vi "input (SubVI).vi"(11 "Controller_NUC":sgl[](array[numeric])) -> (3 "Controller Input":T1 {"Joy1 Y-axis" scale=-32767.0..32767.0; "Joy2 Y-axis" scale=-32767.0..32767.0; "Joy2 X-axis" scale=-32767.0..32767.0; "Joy1 X-axis" scale=-32767.0..32767.0; "Z axis - LT~RT" scale=-32767.0..32767.0; "DPad" scale=0.0..360.0})   [LabVIEW 2016]
uses:
  YSH_XBOX360_joystick.ctl
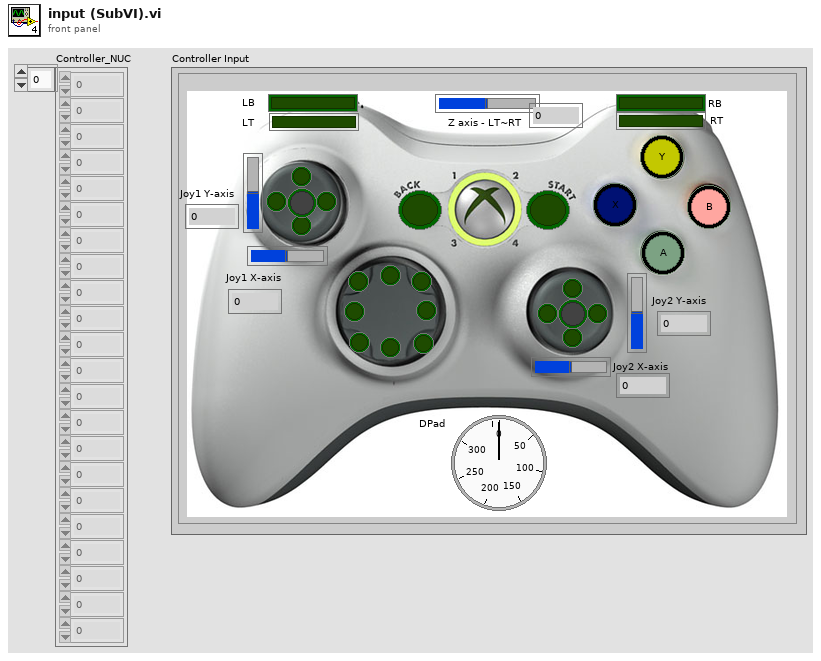
[diagram p1: front panel]
types:
  T1 = typedef "YSH_XBOX360_joystick.ctl" = cluster{"RR":bool, "RL":bool, "RD":bool, "RU":bool, "LR":bool, "LL":bool, "LD":bool, "LU":bool, "Back":bool, "Start":bool, "DPad":dbl, "D Pad":cluster{"0":bool, "45":bool, "90":bool, "135":bool, "180":bool, "215":bool, "270":bool, "315":bool}, "A":bool, "B":bool, "X":bool, "Y":bool, "LB":bool, "RB":bool, "LT":bool, "RT":bool, "Left Joy Push":bool, "Right Joy Push":bool, "Z axis - LT~RT":i32, "Joy1 X-axis":i32, "Joy2 X-axis":i32, "Joy2 Y-axis":i32, "Joy1 Y-axis":i32}
  T2 = cluster{"[0]":bool, "[1]":bool, "[2]":bool, "[3]":bool, "[4]":bool, "[5]":bool, "[6]":bool, "[7]":bool}
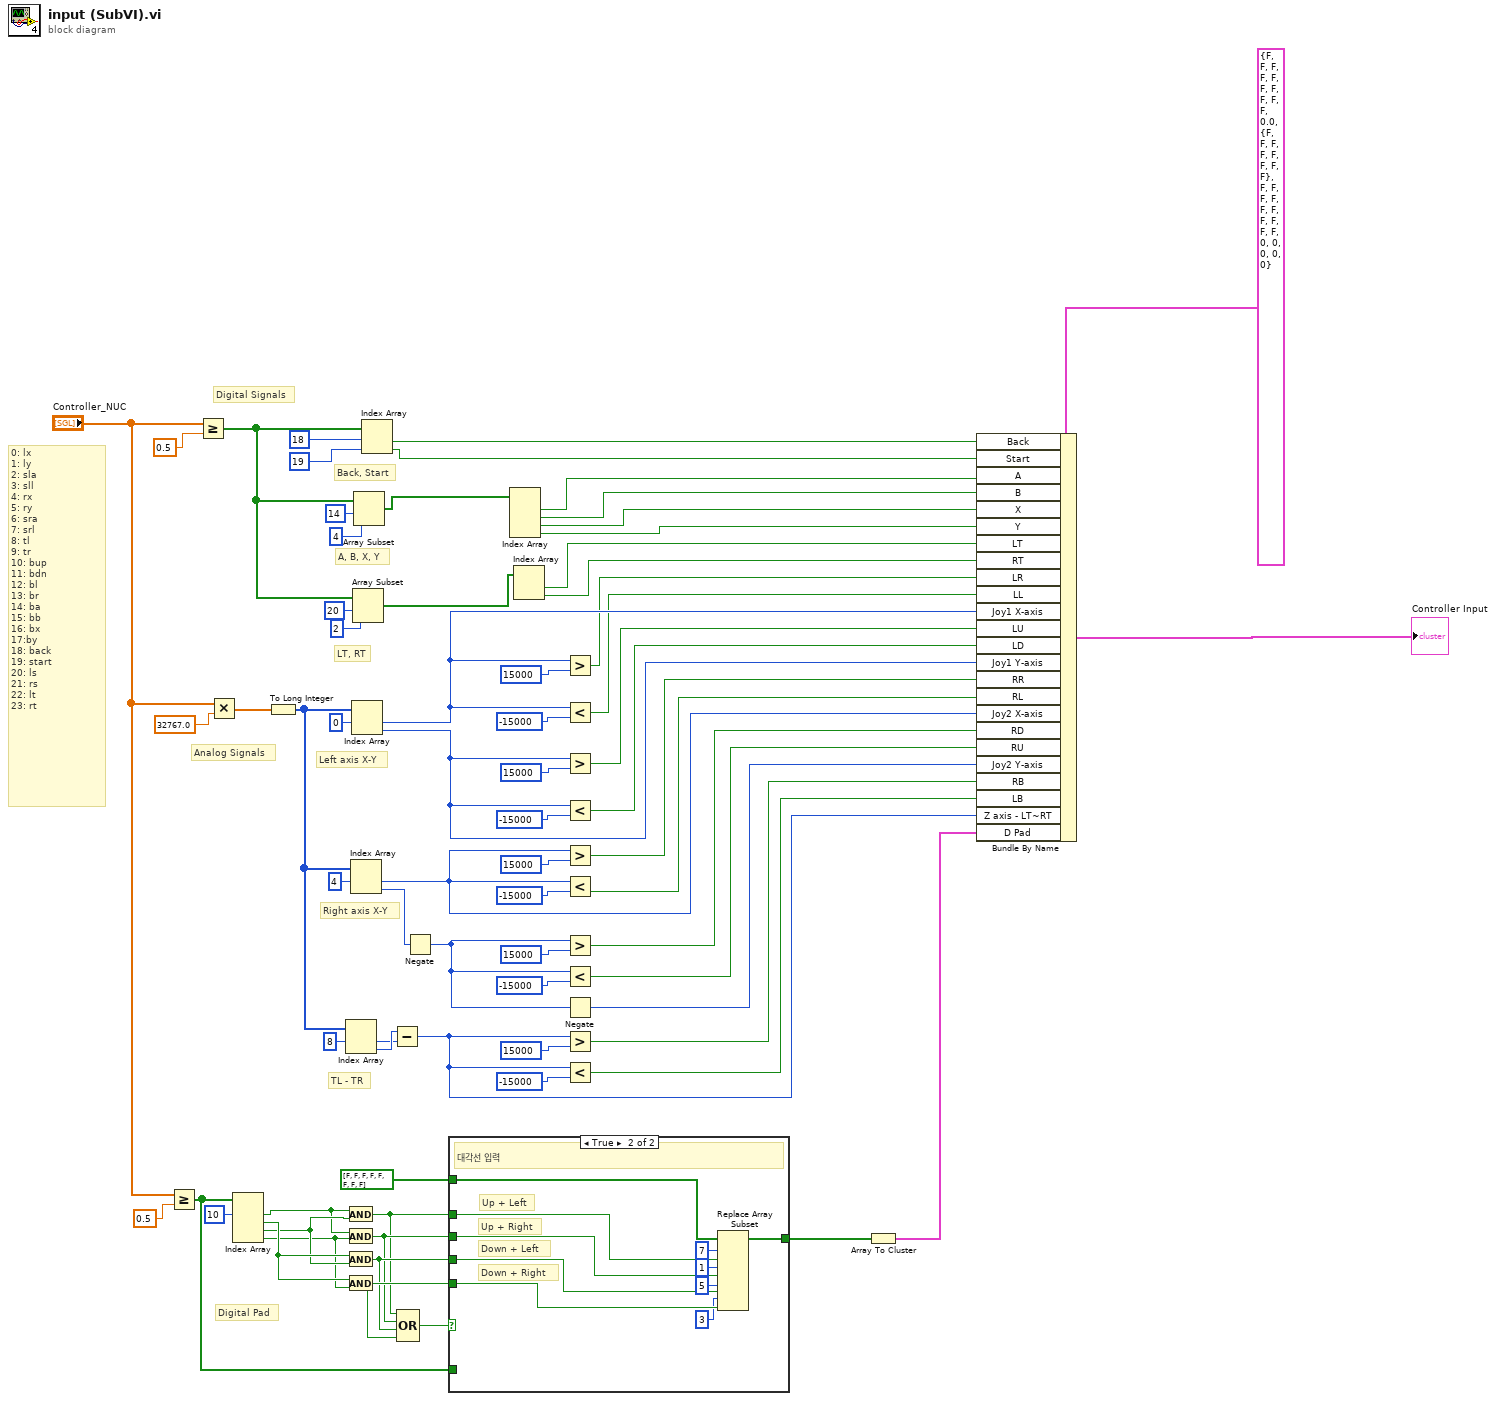
[diagram p0: block diagram]
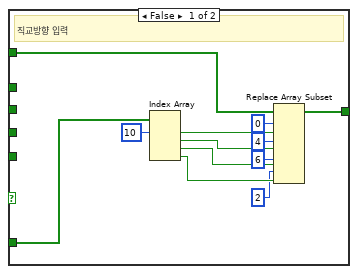
[diagram p2: hidden frame]
diagram:
  # "Analog Signals"
  # "Digital Pad"
  # "TL - TR"
  # "Right axis X-Y"
  # "Left axis X-Y"
  # "LT, RT"
  # "A, B, X, Y"
  # "Back, Start"
  # "Digital Signals"
  # "0: lx\n1: ly\n2: sla\n3: sll\n4: rx\n5: ry\n6: sra\n7: srl\n8: tl\n9: tr\n10: bup\n11: bdn\n12: bl\n13: br\n14: ba\n15: bb\n16: bx\n17:by\n18: back\n19: start\n20: ls\n21: rs\n22: lt\n23: rt"
  n1 = Greater Or Equal?(x="Controller_NUC", y=sgl 0.5) -> (x >= y?=w59:bool[])
  n2 = Greater Or Equal?(x="Controller_NUC", y=sgl 0.5) -> (x >= y?=w13:bool[])
  n3 = Multiply(x="Controller_NUC", y=sgl 32767.0) -> (x*y=w22:sgl[])
  n4 = Index Array(array=w59, index #1=10 ("인덱스")) -> (element #1=w68:bool, element #2=w71:bool, element #3=w70:bool, element #4=w69:bool)  [unwired: 3 in]
  n5 = To Long Integer(number=w22) -> (32bit integer=w48:i32[])
  n6 = Index Array(array=w48, index #1=8 ("인덱스")) -> (element #1=w49:i32, element #2=w50:i32)  [unwired: 1 in]
  n7 = And(x=w68, y=w70) -> (x .and. y?=w61:bool)
  n8 = And(x=w68, y=w69) -> (x .and. y?=w62:bool)
  n9 = And(x=w71, y=w70) -> (x .and. y?=w63:bool)
  n10 = And(x=w71, y=w69) -> (x .and. y?=w64:bool)
  n11 = Index Array(array=w48, index #1=4 ("인덱스")) -> (element #1=w41:i32, element #2=w42:i32)  [unwired: 1 in]
  n12 = Index Array(array=w48, index #1=0 ("인덱스")) -> (element #1=w28:i32, element #2=w33:i32)  [unwired: 1 in]
  n13 = Array Subset(array=w13, index=20 ("인덱스"), length=2 ("길이")) -> (w16:bool[])
  n14 = Array Subset(array=w13, index=14 ("인덱스"), length=4 ("길이")) -> (w8:bool[])
  n15 = Index Array(array=w13, index #1=18 ("인덱스"), index #2=19 ("인덱스")) -> (element #1=w3:bool, element #2=w4:bool)
  n16 = Subtract(x=w50, y=w49) -> (x-y=w55:i32)
  n17 = Compound Arithmetic op=OR(w61, w62, w63, w64) -> (w60:bool)
  n18 = Negate(x=w42) -> (-x=w45:i32)
  n19 = case shown="True" w60 {
    tunnel: bool[] [FALSE, FALSE, FALSE, FALSE, FALSE, FALSE, FALSE, FALSE] -> [w83 w93]
    tunnel: [w82 w92] -> w66
    tunnel: w59 -> [w80 _]
    tunnel: w61 -> [_ w91]
    tunnel: w62 -> [_ w90]
    tunnel: w63 -> [_ w89]
    tunnel: w64 -> [_ w88]
    frame False {
      # "직교방향 입력"
      n20 = Index Array(array=w80, index #1=10 ("인덱스")) -> (element #1=w79:bool, element #2=w78:bool, element #3=w77:bool, element #4=w76:bool)  [unwired: 3 in]
      n21 = Replace Array Subset(array=w83, new element #1=w79, index #1=0 ("인덱스"), new element #2=w78, index #2=4 ("인덱스"), new element #3=w77, index #3=6 ("인덱스"), new element #4=w76, index #4=2 ("인덱스")) -> (w82:bool[])
    }
    frame True {
      # "Up + Right"
      # "Down + Right"
      # "Down + Left"
      # "Up + Left"
      # "대각선 입력"
      n22 = Replace Array Subset(array=w93, new element #1=w91, index #1=7 ("인덱스"), new element #2=w90, index #2=1 ("인덱스"), new element #3=w89, index #3=5 ("인덱스"), new element #4=w88, index #4=3 ("인덱스")) -> (w92:bool[])
    }
  }
  n23 = Index Array(array=w8) -> (element #1=w9:bool, element #2=w10:bool, element #3=w11:bool, element #4=w12:bool)  [unwired: 4 in]
  n24 = Index Array(array=w16) -> (element #1=w17:bool, element #2=w18:bool)  [unwired: 2 in]
  n25 = Greater?(x=w28, y=15000) -> (0:w26:bool)
  n26 = Less?(x=w28, y=-15000) -> (x < y?=w27:bool)
  n27 = Greater?(x=w33, y=15000) -> (0:w31:bool)
  n28 = Less?(x=w33, y=-15000) -> (x < y?=w32:bool)
  n29 = Greater?(x=w41, y=15000) -> (0:w39:bool)
  n30 = Less?(x=w41, y=-15000) -> (x < y?=w40:bool)
  n31 = Greater?(x=w45, y=15000) -> (0:w43:bool)
  n32 = Less?(x=w45, y=-15000) -> (x < y?=w44:bool)
  n33 = Negate(x=w45) -> (-x=w46:i32)
  n34 = Greater?(x=w55, y=15000) -> (0:w53:bool)
  n35 = Less?(x=w55, y=-15000) -> (x < y?=w54:bool)
  n36 = Array To Cluster(array=w66) -> (cluster=w67:T2)
  n37 = Bundle By Name(cluster=T1 {"RR"=FALSE, "RL"=FALSE, "RD"=FALSE, "RU"=FALSE, "LR"=FALSE, "LL"=FALSE, "LD"=FALSE, "LU"=FALSE, "Back"=FALSE, "Start"=FALSE, "DPad"=0.0, "D Pad"={"0"=FALSE, "45"=FALSE, "90"=FALSE, "135"=FALSE, "180"=FALSE, "215"=FALSE, "270"=FALSE, "315"=FALSE}, "A"=FALSE, "B"=FALSE, "X"=FALSE, "Y"=FALSE, "LB"=FALSE, "RB"=FALSE, "LT"=FALSE, "RT"=FALSE, "Left Joy Push"=FALSE, "Right Joy Push"=FALSE, "Z axis - LT~RT"=0, "Joy1 X-axis"=0, "Joy2 X-axis"=0, "Joy2 Y-axis"=0, "Joy1 Y-axis"=0} ("Controller Input"), "Back"=w3, "Start"=w4, "A"=w9, "B"=w10, "X"=w11, "Y"=w12, "LT"=w17, "RT"=w18, "LR"=w26, "LL"=w27, "Joy1 X-axis"=w28, "LU"=w31, "LD"=w32, "Joy1 Y-axis"=w33, "RR"=w39, "RL"=w40, "Joy2 X-axis"=w41, "RD"=w43, "RU"=w44, "Joy2 Y-axis"=w46, "RB"=w53, "LB"=w54, "Z axis - LT~RT"=w55, "D Pad"=w67) -> (→"Controller Input":T1)
